vi "GE 5565PIORC.PIO.Array.vi"(10 "count (100)":i32=100, 11 "data type":T1) -> (0 "error out":errorcluster, 3 "pass?":bool)   [LabVIEW 2020]
uses:
  Typedefs/GE 5565PIORC.Data Types.ctl
  Source/GE 5565PIORC.lvclass/GE 5565PIORC.ctl
  Source/Methods/GE 5565PIORC.PIO.Write (1D Bool).vi
  Source/Methods/GE 5565PIORC.PIO.Read (1D Bool).vi
  Source/Methods/GE 5565PIORC.PIO.Write (1D SGL).vi
  Source/Methods/GE 5565PIORC.PIO.Read (1D SGL).vi
  Source/Methods/GE 5565PIORC.PIO.Write (1D DBL).vi
  Source/Methods/GE 5565PIORC.PIO.Read (1D DBL).vi
  Source/Methods/GE 5565PIORC.PIO.Write (1D I8).vi
  Source/Methods/GE 5565PIORC.PIO.Read (1D I8).vi
  Source/Methods/GE 5565PIORC.PIO.Write (1D I16).vi
  Source/Methods/GE 5565PIORC.PIO.Read (1D I16).vi
  Source/Methods/GE 5565PIORC.PIO.Write (1D I32).vi
  Source/Methods/GE 5565PIORC.PIO.Read (1D I32).vi
  Source/Methods/GE 5565PIORC.PIO.Write (1D I64).vi
  Source/Methods/GE 5565PIORC.PIO.Read (1D I64).vi
  Source/Methods/GE 5565PIORC.PIO.Write (1D U8).vi
  Source/Methods/GE 5565PIORC.PIO.Read (1D U8).vi
  Source/Methods/GE 5565PIORC.PIO.Write (1D U16).vi
  Source/Methods/GE 5565PIORC.PIO.Read (1D U16).vi
  Source/Methods/GE 5565PIORC.PIO.Write (1D U32).vi
  Source/Methods/GE 5565PIORC.PIO.Read (1D U32).vi
  Source/Methods/GE 5565PIORC.PIO.Write (1D U64).vi
  Source/Methods/GE 5565PIORC.PIO.Read (1D U64).vi
  Source/Methods/GE 5565PIORC.VISA.Move Out.vi
  Source/Methods/GE 5565PIORC.VISA.Move Out.String (U8).vi
  Source/Methods/GE 5565PIORC.VISA.Move In.vi
  Source/Methods/GE 5565PIORC.VISA.Move In.String (U8).vi
  Source/Methods/GE 5565PIORC.VISA.Return Handler.vi
  <vilib>/Utility/error.llb/Error Cluster From Error Code.vi
  Source/GE 5565PIORC.lvclass
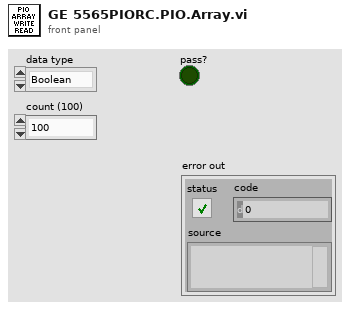
[diagram p1: front panel]
types:
  T1 = typedef "GE 5565PIORC.Data Types.ctl" = enum16{"Boolean", "Single", "Double", "I8", "I16", "I32", "I64", "U8", "U16", "U32", "U64"}
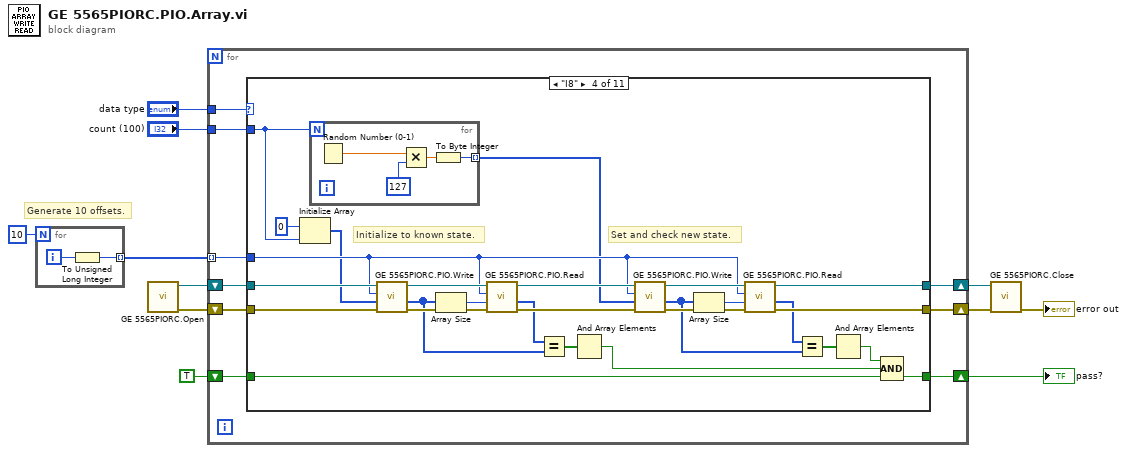
[diagram p0: block diagram]
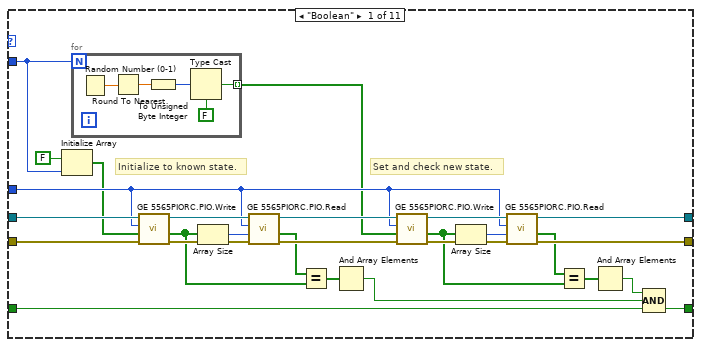
[diagram p2: hidden frame]
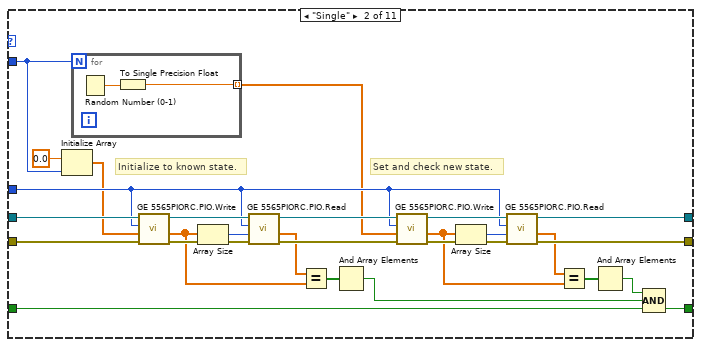
[diagram p3: hidden frame]
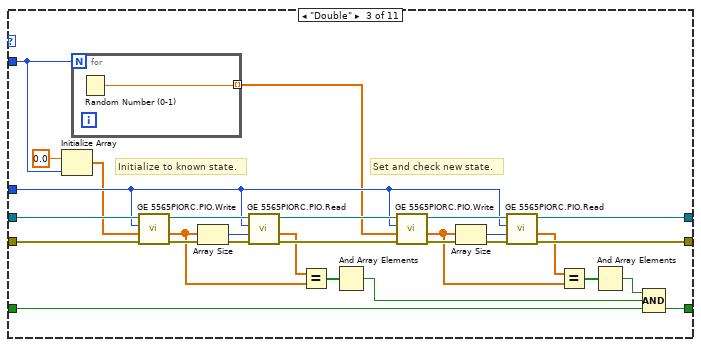
[diagram p4: hidden frame]
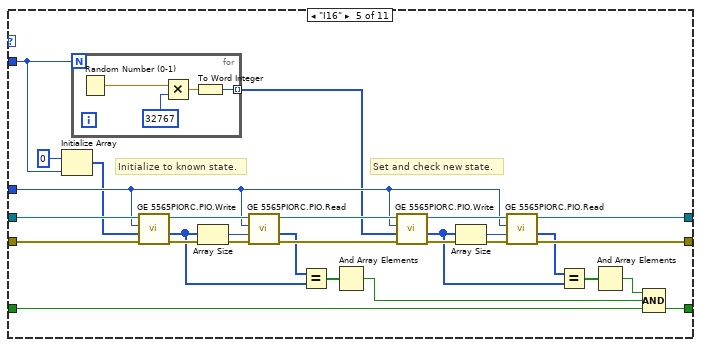
[diagram p5: hidden frame]
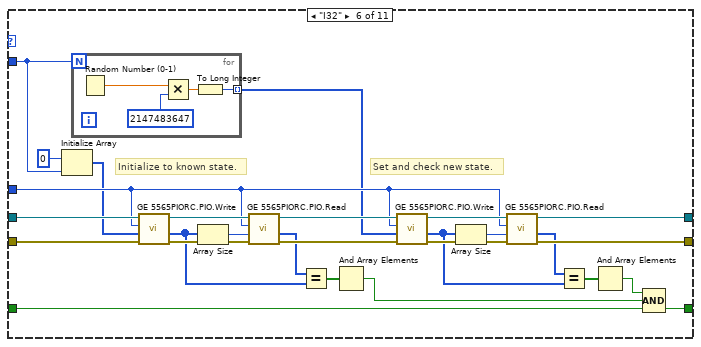
[diagram p6: hidden frame]
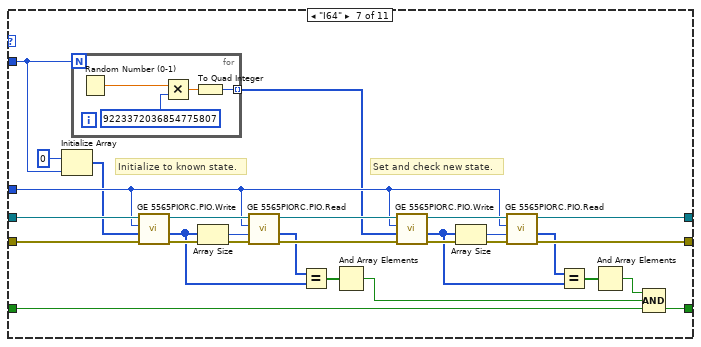
[diagram p7: hidden frame]
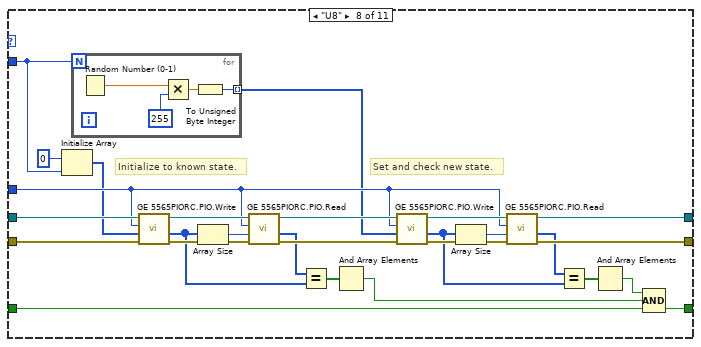
[diagram p8: hidden frame]
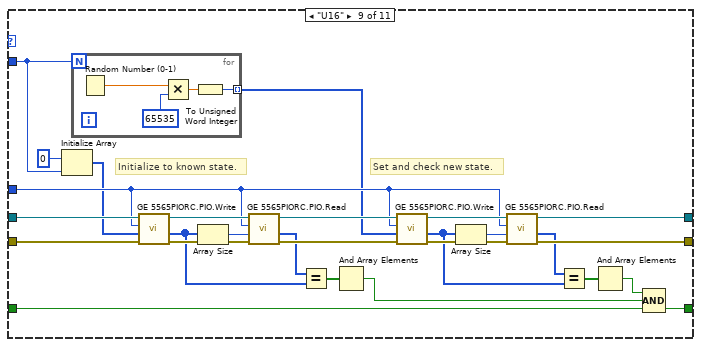
[diagram p9: hidden frame]
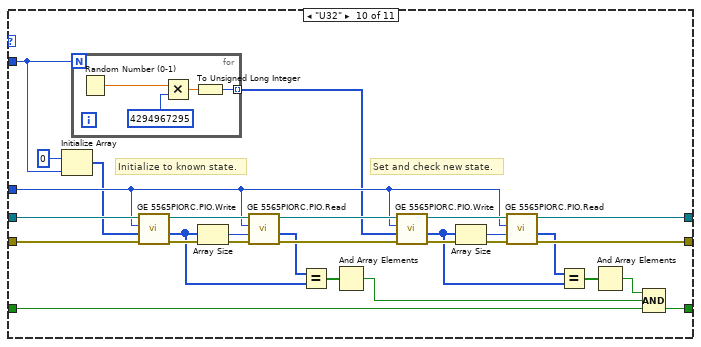
[diagram p10: hidden frame]
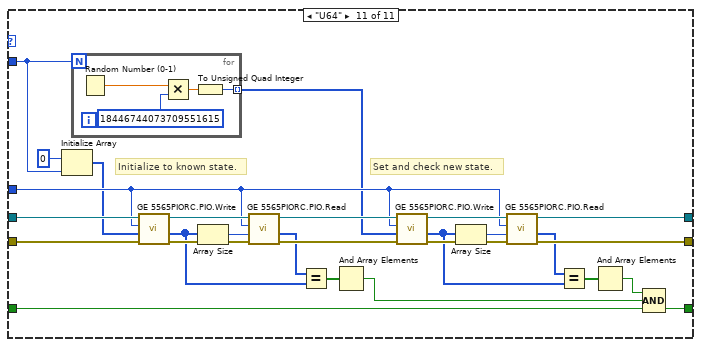
[diagram p11: hidden frame]
diagram:
  # "Generate 10 offsets."
  n1 = for {
    N: 10 -> [_]
    tunnel: [w13] -> w10 mode=indexing
    i -> [w12]
    n2 = To Unsigned Long Integer(number=w12) -> (unsigned 32bit integer=w13:u32)
  }
  n3 = call "GE 5565PIORC.Open.vi"() -> ("error out"=w6:errorcluster, "GE 5565PIORC"=w5:refnum<class "GE 5565PIORC.lvclass">)  [unwired: 10 in]
  n4 = for {
    tunnel: w10 -> [w21] mode=indexing
    tunnel: "data type" -> [w20]
    shift-right: [w16] -> w4
    shift-left: w5 -> [w22]
    shift-right: [w15] -> w3
    shift-left: w6 -> [w19]
    shift-right: [w17] -> w7
    shift-left: TRUE -> [w18]
    tunnel: "count (100)" -> [w14]
    n5 = case shown="\"I8\"" w20 {
      tunnel: w22 -> [w49 w81 w110 w138 w169 w200 w231 w262 w293 w324 w355]
      tunnel: w21 -> [w33 w65 w94 w122 w153 w184 w215 w246 w277 w308 w339]
      tunnel: w19 -> [w48 w80 w109 w137 w168 w199 w230 w261 w292 w323 w354]
      tunnel: w18 -> [w43 w75 w104 w132 w163 w194 w225 w256 w287 w318 w349]
      tunnel: [w42 w74 w103 w131 w162 w193 w224 w255 w286 w317 w348] -> w17
      tunnel: [w41 w73 w102 w130 w161 w192 w223 w254 w285 w316 w347] -> w16
      tunnel: [w40 w72 w101 w129 w160 w191 w222 w253 w284 w315 w346] -> w15
      tunnel: w14 -> [w29 w61 w90 w118 w149 w180 w211 w242 w273 w304 w335]
      frame "Boolean" {
        # "Set and check new state."
        # "Initialize to known state."
        n6 = Initialize Array(FALSE ("data"), w29) -> (w30:bool[])
        n7 = for {
          N: w29 -> [_]
          tunnel: [w50] -> w28 mode=indexing
          n8 = Random Number (0-1)() -> (number: 0 to 1=w54:dbl)
          n9 = Round To Nearest(number=w54) -> (nearest integer value=w53:dbl)
          n10 = To Unsigned Byte Integer(number=w53) -> (unsigned 8bit integer=w52:u8)
          n11 = Type Cast(type=FALSE, x=w52) -> (*(type *) &x=w50:bool)
        }
        n12 = call-poly "GE 5565PIORC.PIO.Write.vi"("error in (no error)"=w48, "data"=w30, "offset"=w33, "GE 5565PIORC in"=w49) -> ("error out"=w46:errorcluster, "data out"=w27:bool[], "GE 5565PIORC out"=w47:refnum<class "GE 5565PIORC.lvclass">)  [unwired: 5 in]
        n13 = Array Size(array=w27) -> (size(s)=w26:i32)
        n14 = call-poly "GE 5565PIORC.PIO.Read.vi"("error in (no error)"=w46, "count"=w26, "offset"=w33, "GE 5565PIORC in"=w47) -> ("error out"=w45:errorcluster, "data"=w39:bool[], "GE 5565PIORC out"=w44:refnum<class "GE 5565PIORC.lvclass">)  [unwired: 5 in]
        n15 = Equal?(x=w39, y=w27) -> (x = y?=w35:bool[])
        n16 = And Array Elements(Boolean array=w35) -> (logical AND=w32:bool)
        n17 = call-poly "GE 5565PIORC.PIO.Write.vi"("error in (no error)"=w45, "data"=w28, "offset"=w33, "GE 5565PIORC in"=w44) -> ("error out"=w37:errorcluster, "data out"=w25:bool[], "GE 5565PIORC out"=w38:refnum<class "GE 5565PIORC.lvclass">)  [unwired: 5 in]
        n18 = Array Size(array=w25) -> (size(s)=w24:i32)
        n19 = call-poly "GE 5565PIORC.PIO.Read.vi"("error in (no error)"=w37, "count"=w24, "offset"=w33, "GE 5565PIORC in"=w38) -> ("error out"=w40:errorcluster, "data"=w36:bool[], "GE 5565PIORC out"=w41:refnum<class "GE 5565PIORC.lvclass">)  [unwired: 5 in]
        n20 = Equal?(x=w36, y=w25) -> (x = y?=w34:bool[])
        n21 = And Array Elements(Boolean array=w34) -> (logical AND=w23:bool)
        n22 = Compound Arithmetic op=AND(w23, w32, w43) -> (w42:bool)
      }
      frame "Single" {
        # "Set and check new state."
        # "Initialize to known state."
        n23 = Initialize Array(sgl 0.0 ("data"), w61) -> (w62:sgl[])
        n24 = for {
          N: w61 -> [_]
          tunnel: [w82] -> w60 mode=indexing
          n25 = Random Number (0-1)() -> (number: 0 to 1=w83:dbl)
          n26 = To Single Precision Float(number=w83) -> (single precision float=w82:sgl)
        }
        n27 = call-poly "GE 5565PIORC.PIO.Write.vi"("error in (no error)"=w80, "data"=w62, "offset"=w65, "GE 5565PIORC in"=w81) -> ("error out"=w78:errorcluster, "data out"=w59:sgl[], "GE 5565PIORC out"=w79:refnum<class "GE 5565PIORC.lvclass">)  [unwired: 5 in]
        n28 = Array Size(array=w59) -> (size(s)=w58:i32)
        n29 = call-poly "GE 5565PIORC.PIO.Read.vi"("error in (no error)"=w78, "count"=w58, "offset"=w65, "GE 5565PIORC in"=w79) -> ("error out"=w77:errorcluster, "data"=w71:sgl[], "GE 5565PIORC out"=w76:refnum<class "GE 5565PIORC.lvclass">)  [unwired: 5 in]
        n30 = Equal?(x=w71, y=w59) -> (x = y?=w67:bool[])
        n31 = And Array Elements(Boolean array=w67) -> (logical AND=w64:bool)
        n32 = call-poly "GE 5565PIORC.PIO.Write.vi"("error in (no error)"=w77, "data"=w60, "offset"=w65, "GE 5565PIORC in"=w76) -> ("error out"=w69:errorcluster, "data out"=w57:sgl[], "GE 5565PIORC out"=w70:refnum<class "GE 5565PIORC.lvclass">)  [unwired: 5 in]
        n33 = Array Size(array=w57) -> (size(s)=w56:i32)
        n34 = call-poly "GE 5565PIORC.PIO.Read.vi"("error in (no error)"=w69, "count"=w56, "offset"=w65, "GE 5565PIORC in"=w70) -> ("error out"=w72:errorcluster, "data"=w68:sgl[], "GE 5565PIORC out"=w73:refnum<class "GE 5565PIORC.lvclass">)  [unwired: 5 in]
        n35 = Equal?(x=w68, y=w57) -> (x = y?=w66:bool[])
        n36 = And Array Elements(Boolean array=w66) -> (logical AND=w55:bool)
        n37 = Compound Arithmetic op=AND(w55, w64, w75) -> (w74:bool)
      }
      frame "Double" {
        # "Set and check new state."
        # "Initialize to known state."
        n38 = Initialize Array(0.0 ("data"), w90) -> (w91:dbl[])
        n39 = for {
          N: w90 -> [_]
          tunnel: [w111] -> w89 mode=indexing
          n40 = Random Number (0-1)() -> (number: 0 to 1=w111:dbl)
        }
        n41 = call-poly "GE 5565PIORC.PIO.Write.vi"("error in (no error)"=w109, "data"=w91, "offset"=w94, "GE 5565PIORC in"=w110) -> ("error out"=w107:errorcluster, "data out"=w88:dbl[], "GE 5565PIORC out"=w108:refnum<class "GE 5565PIORC.lvclass">)  [unwired: 5 in]
        n42 = Array Size(array=w88) -> (size(s)=w87:i32)
        n43 = call-poly "GE 5565PIORC.PIO.Read.vi"("error in (no error)"=w107, "count"=w87, "offset"=w94, "GE 5565PIORC in"=w108) -> ("error out"=w106:errorcluster, "data"=w100:dbl[], "GE 5565PIORC out"=w105:refnum<class "GE 5565PIORC.lvclass">)  [unwired: 5 in]
        n44 = Equal?(x=w100, y=w88) -> (x = y?=w96:bool[])
        n45 = And Array Elements(Boolean array=w96) -> (logical AND=w93:bool)
        n46 = call-poly "GE 5565PIORC.PIO.Write.vi"("error in (no error)"=w106, "data"=w89, "offset"=w94, "GE 5565PIORC in"=w105) -> ("error out"=w98:errorcluster, "data out"=w86:dbl[], "GE 5565PIORC out"=w99:refnum<class "GE 5565PIORC.lvclass">)  [unwired: 5 in]
        n47 = Array Size(array=w86) -> (size(s)=w85:i32)
        n48 = call-poly "GE 5565PIORC.PIO.Read.vi"("error in (no error)"=w98, "count"=w85, "offset"=w94, "GE 5565PIORC in"=w99) -> ("error out"=w101:errorcluster, "data"=w97:dbl[], "GE 5565PIORC out"=w102:refnum<class "GE 5565PIORC.lvclass">)  [unwired: 5 in]
        n49 = Equal?(x=w97, y=w86) -> (x = y?=w95:bool[])
        n50 = And Array Elements(Boolean array=w95) -> (logical AND=w84:bool)
        n51 = Compound Arithmetic op=AND(w84, w93, w104) -> (w103:bool)
      }
      frame "I8" {
        # "Set and check new state."
        # "Initialize to known state."
        n52 = Initialize Array(i8 0 ("data"), w118) -> (w119:i8[])
        n53 = for {
          N: w118 -> [_]
          tunnel: [w139] -> w117 mode=indexing
          n54 = Random Number (0-1)() -> (number: 0 to 1=w142:dbl)
          n55 = Multiply(x=w142, y=i8 127) -> (x*y=w140:dbl)
          n56 = To Byte Integer(number=w140) -> (8bit integer=w139:i8)
        }
        n57 = call-poly "GE 5565PIORC.PIO.Write.vi"("error in (no error)"=w137, "data"=w119, "offset"=w122, "GE 5565PIORC in"=w138) -> ("error out"=w135:errorcluster, "data out"=w116:i8[], "GE 5565PIORC out"=w136:refnum<class "GE 5565PIORC.lvclass">)  [unwired: 5 in]
        n58 = Array Size(array=w116) -> (size(s)=w115:i32)
        n59 = call-poly "GE 5565PIORC.PIO.Read.vi"("error in (no error)"=w135, "count"=w115, "offset"=w122, "GE 5565PIORC in"=w136) -> ("error out"=w134:errorcluster, "data"=w128:i8[], "GE 5565PIORC out"=w133:refnum<class "GE 5565PIORC.lvclass">)  [unwired: 5 in]
        n60 = Equal?(x=w128, y=w116) -> (x = y?=w124:bool[])
        n61 = And Array Elements(Boolean array=w124) -> (logical AND=w121:bool)
        n62 = call-poly "GE 5565PIORC.PIO.Write.vi"("error in (no error)"=w134, "data"=w117, "offset"=w122, "GE 5565PIORC in"=w133) -> ("error out"=w126:errorcluster, "data out"=w114:i8[], "GE 5565PIORC out"=w127:refnum<class "GE 5565PIORC.lvclass">)  [unwired: 5 in]
        n63 = Array Size(array=w114) -> (size(s)=w113:i32)
        n64 = call-poly "GE 5565PIORC.PIO.Read.vi"("error in (no error)"=w126, "count"=w113, "offset"=w122, "GE 5565PIORC in"=w127) -> ("error out"=w129:errorcluster, "data"=w125:i8[], "GE 5565PIORC out"=w130:refnum<class "GE 5565PIORC.lvclass">)  [unwired: 5 in]
        n65 = Equal?(x=w125, y=w114) -> (x = y?=w123:bool[])
        n66 = And Array Elements(Boolean array=w123) -> (logical AND=w112:bool)
        n67 = Compound Arithmetic op=AND(w112, w121, w132) -> (w131:bool)
      }
      frame "I16" {
        # "Set and check new state."
        # "Initialize to known state."
        n68 = Initialize Array(i16 0 ("data"), w149) -> (w150:i16[])
        n69 = for {
          N: w149 -> [_]
          tunnel: [w170] -> w148 mode=indexing
          n70 = Random Number (0-1)() -> (number: 0 to 1=w173:dbl)
          n71 = Multiply(x=w173, y=i16 32767) -> (x*y=w171:dbl)
          n72 = To Word Integer(number=w171) -> (16bit integer=w170:i16)
        }
        n73 = call-poly "GE 5565PIORC.PIO.Write.vi"("error in (no error)"=w168, "data"=w150, "offset"=w153, "GE 5565PIORC in"=w169) -> ("error out"=w166:errorcluster, "data out"=w147:i16[], "GE 5565PIORC out"=w167:refnum<class "GE 5565PIORC.lvclass">)  [unwired: 5 in]
        n74 = Array Size(array=w147) -> (size(s)=w146:i32)
        n75 = call-poly "GE 5565PIORC.PIO.Read.vi"("error in (no error)"=w166, "count"=w146, "offset"=w153, "GE 5565PIORC in"=w167) -> ("error out"=w165:errorcluster, "data"=w159:i16[], "GE 5565PIORC out"=w164:refnum<class "GE 5565PIORC.lvclass">)  [unwired: 5 in]
        n76 = Equal?(x=w159, y=w147) -> (x = y?=w155:bool[])
        n77 = And Array Elements(Boolean array=w155) -> (logical AND=w152:bool)
        n78 = call-poly "GE 5565PIORC.PIO.Write.vi"("error in (no error)"=w165, "data"=w148, "offset"=w153, "GE 5565PIORC in"=w164) -> ("error out"=w157:errorcluster, "data out"=w145:i16[], "GE 5565PIORC out"=w158:refnum<class "GE 5565PIORC.lvclass">)  [unwired: 5 in]
        n79 = Array Size(array=w145) -> (size(s)=w144:i32)
        n80 = call-poly "GE 5565PIORC.PIO.Read.vi"("error in (no error)"=w157, "count"=w144, "offset"=w153, "GE 5565PIORC in"=w158) -> ("error out"=w160:errorcluster, "data"=w156:i16[], "GE 5565PIORC out"=w161:refnum<class "GE 5565PIORC.lvclass">)  [unwired: 5 in]
        n81 = Equal?(x=w156, y=w145) -> (x = y?=w154:bool[])
        n82 = And Array Elements(Boolean array=w154) -> (logical AND=w143:bool)
        n83 = Compound Arithmetic op=AND(w143, w152, w163) -> (w162:bool)
      }
      frame "I32" {
        # "Set and check new state."
        # "Initialize to known state."
        n84 = Initialize Array(0 ("data"), w180) -> (w181:i32[])
        n85 = for {
          N: w180 -> [_]
          tunnel: [w201] -> w179 mode=indexing
          n86 = Random Number (0-1)() -> (number: 0 to 1=w204:dbl)
          n87 = Multiply(x=w204, y=2147483647) -> (x*y=w202:dbl)
          n88 = To Long Integer(number=w202) -> (32bit integer=w201:i32)
        }
        n89 = call-poly "GE 5565PIORC.PIO.Write.vi"("error in (no error)"=w199, "data"=w181, "offset"=w184, "GE 5565PIORC in"=w200) -> ("error out"=w197:errorcluster, "data out"=w178:i32[], "GE 5565PIORC out"=w198:refnum<class "GE 5565PIORC.lvclass">)  [unwired: 5 in]
        n90 = Array Size(array=w178) -> (size(s)=w177:i32)
        n91 = call-poly "GE 5565PIORC.PIO.Read.vi"("error in (no error)"=w197, "count"=w177, "offset"=w184, "GE 5565PIORC in"=w198) -> ("error out"=w196:errorcluster, "data"=w190:i32[], "GE 5565PIORC out"=w195:refnum<class "GE 5565PIORC.lvclass">)  [unwired: 5 in]
        n92 = Equal?(x=w190, y=w178) -> (x = y?=w186:bool[])
        n93 = And Array Elements(Boolean array=w186) -> (logical AND=w183:bool)
        n94 = call-poly "GE 5565PIORC.PIO.Write.vi"("error in (no error)"=w196, "data"=w179, "offset"=w184, "GE 5565PIORC in"=w195) -> ("error out"=w188:errorcluster, "data out"=w176:i32[], "GE 5565PIORC out"=w189:refnum<class "GE 5565PIORC.lvclass">)  [unwired: 5 in]
        n95 = Array Size(array=w176) -> (size(s)=w175:i32)
        n96 = call-poly "GE 5565PIORC.PIO.Read.vi"("error in (no error)"=w188, "count"=w175, "offset"=w184, "GE 5565PIORC in"=w189) -> ("error out"=w191:errorcluster, "data"=w187:i32[], "GE 5565PIORC out"=w192:refnum<class "GE 5565PIORC.lvclass">)  [unwired: 5 in]
        n97 = Equal?(x=w187, y=w176) -> (x = y?=w185:bool[])
        n98 = And Array Elements(Boolean array=w185) -> (logical AND=w174:bool)
        n99 = Compound Arithmetic op=AND(w174, w183, w194) -> (w193:bool)
      }
      frame "I64" {
        # "Set and check new state."
        # "Initialize to known state."
        n100 = Initialize Array(i64 0 ("data"), w211) -> (w212:i64[])
        n101 = for {
          N: w211 -> [_]
          tunnel: [w232] -> w210 mode=indexing
          n102 = Random Number (0-1)() -> (number: 0 to 1=w235:dbl)
          n103 = Multiply(x=w235, y=i64 9223372036854775807) -> (x*y=w233:dbl)
          n104 = To Quad Integer(1:w233) -> (0:w232:i64)
        }
        n105 = call-poly "GE 5565PIORC.PIO.Write.vi"("error in (no error)"=w230, "data"=w212, "offset"=w215, "GE 5565PIORC in"=w231) -> ("error out"=w228:errorcluster, "data out"=w209:i64[], "GE 5565PIORC out"=w229:refnum<class "GE 5565PIORC.lvclass">)  [unwired: 5 in]
        n106 = Array Size(array=w209) -> (size(s)=w208:i32)
        n107 = call-poly "GE 5565PIORC.PIO.Read.vi"("error in (no error)"=w228, "count"=w208, "offset"=w215, "GE 5565PIORC in"=w229) -> ("error out"=w227:errorcluster, "data"=w221:i64[], "GE 5565PIORC out"=w226:refnum<class "GE 5565PIORC.lvclass">)  [unwired: 5 in]
        n108 = Equal?(x=w221, y=w209) -> (x = y?=w217:bool[])
        n109 = And Array Elements(Boolean array=w217) -> (logical AND=w214:bool)
        n110 = call-poly "GE 5565PIORC.PIO.Write.vi"("error in (no error)"=w227, "data"=w210, "offset"=w215, "GE 5565PIORC in"=w226) -> ("error out"=w219:errorcluster, "data out"=w207:i64[], "GE 5565PIORC out"=w220:refnum<class "GE 5565PIORC.lvclass">)  [unwired: 5 in]
        n111 = Array Size(array=w207) -> (size(s)=w206:i32)
        n112 = call-poly "GE 5565PIORC.PIO.Read.vi"("error in (no error)"=w219, "count"=w206, "offset"=w215, "GE 5565PIORC in"=w220) -> ("error out"=w222:errorcluster, "data"=w218:i64[], "GE 5565PIORC out"=w223:refnum<class "GE 5565PIORC.lvclass">)  [unwired: 5 in]
        n113 = Equal?(x=w218, y=w207) -> (x = y?=w216:bool[])
        n114 = And Array Elements(Boolean array=w216) -> (logical AND=w205:bool)
        n115 = Compound Arithmetic op=AND(w205, w214, w225) -> (w224:bool)
      }
      frame "U8" {
        # "Set and check new state."
        # "Initialize to known state."
        n116 = Initialize Array(u8 0 ("data"), w242) -> (w243:u8[])
        n117 = for {
          N: w242 -> [_]
          tunnel: [w263] -> w241 mode=indexing
          n118 = Random Number (0-1)() -> (number: 0 to 1=w266:dbl)
          n119 = Multiply(x=w266, y=u8 255) -> (x*y=w264:dbl)
          n120 = To Unsigned Byte Integer(number=w264) -> (unsigned 8bit integer=w263:u8)
        }
        n121 = call-poly "GE 5565PIORC.PIO.Write.vi"("error in (no error)"=w261, "data"=w243, "offset"=w246, "GE 5565PIORC in"=w262) -> ("error out"=w259:errorcluster, "data out"=w240:u8[], "GE 5565PIORC out"=w260:refnum<class "GE 5565PIORC.lvclass">)  [unwired: 5 in]
        n122 = Array Size(array=w240) -> (size(s)=w239:i32)
        n123 = call-poly "GE 5565PIORC.PIO.Read.vi"("error in (no error)"=w259, "count"=w239, "offset"=w246, "GE 5565PIORC in"=w260) -> ("error out"=w258:errorcluster, "data"=w252:u8[], "GE 5565PIORC out"=w257:refnum<class "GE 5565PIORC.lvclass">)  [unwired: 5 in]
        n124 = Equal?(x=w252, y=w240) -> (x = y?=w248:bool[])
        n125 = And Array Elements(Boolean array=w248) -> (logical AND=w245:bool)
        n126 = call-poly "GE 5565PIORC.PIO.Write.vi"("error in (no error)"=w258, "data"=w241, "offset"=w246, "GE 5565PIORC in"=w257) -> ("error out"=w250:errorcluster, "data out"=w238:u8[], "GE 5565PIORC out"=w251:refnum<class "GE 5565PIORC.lvclass">)  [unwired: 5 in]
        n127 = Array Size(array=w238) -> (size(s)=w237:i32)
        n128 = call-poly "GE 5565PIORC.PIO.Read.vi"("error in (no error)"=w250, "count"=w237, "offset"=w246, "GE 5565PIORC in"=w251) -> ("error out"=w253:errorcluster, "data"=w249:u8[], "GE 5565PIORC out"=w254:refnum<class "GE 5565PIORC.lvclass">)  [unwired: 5 in]
        n129 = Equal?(x=w249, y=w238) -> (x = y?=w247:bool[])
        n130 = And Array Elements(Boolean array=w247) -> (logical AND=w236:bool)
        n131 = Compound Arithmetic op=AND(w236, w245, w256) -> (w255:bool)
      }
      frame "U16" {
        # "Set and check new state."
        # "Initialize to known state."
        n132 = Initialize Array(u16 0 ("data"), w273) -> (w274:u16[])
        n133 = for {
          N: w273 -> [_]
          tunnel: [w294] -> w272 mode=indexing
          n134 = Random Number (0-1)() -> (number: 0 to 1=w297:dbl)
          n135 = Multiply(x=w297, y=u16 65535) -> (x*y=w295:dbl)
          n136 = To Unsigned Word Integer(number=w295) -> (unsigned 16bit integer=w294:u16)
        }
        n137 = call-poly "GE 5565PIORC.PIO.Write.vi"("error in (no error)"=w292, "data"=w274, "offset"=w277, "GE 5565PIORC in"=w293) -> ("error out"=w290:errorcluster, "data out"=w271:u16[], "GE 5565PIORC out"=w291:refnum<class "GE 5565PIORC.lvclass">)  [unwired: 5 in]
        n138 = Array Size(array=w271) -> (size(s)=w270:i32)
        n139 = call-poly "GE 5565PIORC.PIO.Read.vi"("error in (no error)"=w290, "count"=w270, "offset"=w277, "GE 5565PIORC in"=w291) -> ("error out"=w289:errorcluster, "data"=w283:u16[], "GE 5565PIORC out"=w288:refnum<class "GE 5565PIORC.lvclass">)  [unwired: 5 in]
        n140 = Equal?(x=w283, y=w271) -> (x = y?=w279:bool[])
        n141 = And Array Elements(Boolean array=w279) -> (logical AND=w276:bool)
        n142 = call-poly "GE 5565PIORC.PIO.Write.vi"("error in (no error)"=w289, "data"=w272, "offset"=w277, "GE 5565PIORC in"=w288) -> ("error out"=w281:errorcluster, "data out"=w269:u16[], "GE 5565PIORC out"=w282:refnum<class "GE 5565PIORC.lvclass">)  [unwired: 5 in]
        n143 = Array Size(array=w269) -> (size(s)=w268:i32)
        n144 = call-poly "GE 5565PIORC.PIO.Read.vi"("error in (no error)"=w281, "count"=w268, "offset"=w277, "GE 5565PIORC in"=w282) -> ("error out"=w284:errorcluster, "data"=w280:u16[], "GE 5565PIORC out"=w285:refnum<class "GE 5565PIORC.lvclass">)  [unwired: 5 in]
        n145 = Equal?(x=w280, y=w269) -> (x = y?=w278:bool[])
        n146 = And Array Elements(Boolean array=w278) -> (logical AND=w267:bool)
        n147 = Compound Arithmetic op=AND(w267, w276, w287) -> (w286:bool)
      }
      frame "U32" {
        # "Set and check new state."
        # "Initialize to known state."
        n148 = Initialize Array(u32 0 ("data"), w304) -> (w305:u32[])
        n149 = for {
          N: w304 -> [_]
          tunnel: [w325] -> w303 mode=indexing
          n150 = Random Number (0-1)() -> (number: 0 to 1=w328:dbl)
          n151 = Multiply(x=w328, y=u32 4294967295) -> (x*y=w326:dbl)
          n152 = To Unsigned Long Integer(number=w326) -> (unsigned 32bit integer=w325:u32)
        }
        n153 = call-poly "GE 5565PIORC.PIO.Write.vi"("error in (no error)"=w323, "data"=w305, "offset"=w308, "GE 5565PIORC in"=w324) -> ("error out"=w321:errorcluster, "data out"=w302:u32[], "GE 5565PIORC out"=w322:refnum<class "GE 5565PIORC.lvclass">)  [unwired: 5 in]
        n154 = Array Size(array=w302) -> (size(s)=w301:i32)
        n155 = call-poly "GE 5565PIORC.PIO.Read.vi"("error in (no error)"=w321, "count"=w301, "offset"=w308, "GE 5565PIORC in"=w322) -> ("error out"=w320:errorcluster, "data"=w314:u32[], "GE 5565PIORC out"=w319:refnum<class "GE 5565PIORC.lvclass">)  [unwired: 5 in]
        n156 = Equal?(x=w314, y=w302) -> (x = y?=w310:bool[])
        n157 = And Array Elements(Boolean array=w310) -> (logical AND=w307:bool)
        n158 = call-poly "GE 5565PIORC.PIO.Write.vi"("error in (no error)"=w320, "data"=w303, "offset"=w308, "GE 5565PIORC in"=w319) -> ("error out"=w312:errorcluster, "data out"=w300:u32[], "GE 5565PIORC out"=w313:refnum<class "GE 5565PIORC.lvclass">)  [unwired: 5 in]
        n159 = Array Size(array=w300) -> (size(s)=w299:i32)
        n160 = call-poly "GE 5565PIORC.PIO.Read.vi"("error in (no error)"=w312, "count"=w299, "offset"=w308, "GE 5565PIORC in"=w313) -> ("error out"=w315:errorcluster, "data"=w311:u32[], "GE 5565PIORC out"=w316:refnum<class "GE 5565PIORC.lvclass">)  [unwired: 5 in]
        n161 = Equal?(x=w311, y=w300) -> (x = y?=w309:bool[])
        n162 = And Array Elements(Boolean array=w309) -> (logical AND=w298:bool)
        n163 = Compound Arithmetic op=AND(w298, w307, w318) -> (w317:bool)
      }
      frame "U64" {
        # "Set and check new state."
        # "Initialize to known state."
        n164 = Initialize Array(u64 0 ("data"), w335) -> (w336:u64[])
        n165 = for {
          N: w335 -> [_]
          tunnel: [w356] -> w334 mode=indexing
          n166 = Random Number (0-1)() -> (number: 0 to 1=w359:dbl)
          n167 = Multiply(x=w359, y=u64 18446744073709551615) -> (x*y=w357:dbl)
          n168 = To Unsigned Quad Integer(1:w357) -> (0:w356:u64)
        }
        n169 = call-poly "GE 5565PIORC.PIO.Write.vi"("error in (no error)"=w354, "data"=w336, "offset"=w339, "GE 5565PIORC in"=w355) -> ("error out"=w352:errorcluster, "data out"=w333:u64[], "GE 5565PIORC out"=w353:refnum<class "GE 5565PIORC.lvclass">)  [unwired: 5 in]
        n170 = Array Size(array=w333) -> (size(s)=w332:i32)
        n171 = call-poly "GE 5565PIORC.PIO.Read.vi"("error in (no error)"=w352, "count"=w332, "offset"=w339, "GE 5565PIORC in"=w353) -> ("error out"=w351:errorcluster, "data"=w345:u64[], "GE 5565PIORC out"=w350:refnum<class "GE 5565PIORC.lvclass">)  [unwired: 5 in]
        n172 = Equal?(x=w345, y=w333) -> (x = y?=w341:bool[])
        n173 = And Array Elements(Boolean array=w341) -> (logical AND=w338:bool)
        n174 = call-poly "GE 5565PIORC.PIO.Write.vi"("error in (no error)"=w351, "data"=w334, "offset"=w339, "GE 5565PIORC in"=w350) -> ("error out"=w343:errorcluster, "data out"=w331:u64[], "GE 5565PIORC out"=w344:refnum<class "GE 5565PIORC.lvclass">)  [unwired: 5 in]
        n175 = Array Size(array=w331) -> (size(s)=w330:i32)
        n176 = call-poly "GE 5565PIORC.PIO.Read.vi"("error in (no error)"=w343, "count"=w330, "offset"=w339, "GE 5565PIORC in"=w344) -> ("error out"=w346:errorcluster, "data"=w342:u64[], "GE 5565PIORC out"=w347:refnum<class "GE 5565PIORC.lvclass">)  [unwired: 5 in]
        n177 = Equal?(x=w342, y=w331) -> (x = y?=w340:bool[])
        n178 = And Array Elements(Boolean array=w340) -> (logical AND=w329:bool)
        n179 = Compound Arithmetic op=AND(w329, w338, w349) -> (w348:bool)
      }
    }
  }
  "pass?" <- w7
  n180 = call "GE 5565PIORC.Close.vi"("error in (no error)"=w3, "GE 5565PIORC"=w4) -> ("error out"=→"error out":errorcluster)  [unwired: 9 in]
